vi "Set-cam-angle.vi"(2 "Rot(CAM)":dbl, 3 "Rot(rad)":dbl) -> (0 "Angle":dbl)   [LabVIEW 2011]
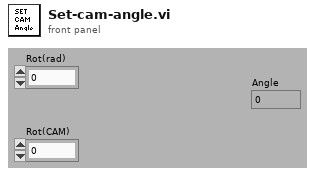
[diagram p1: front panel]
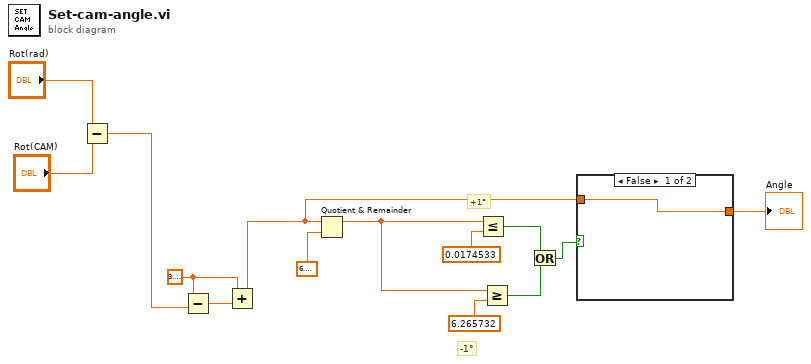
[diagram p0: block diagram]
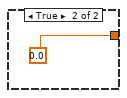
[diagram p2: hidden frame]
diagram:
  w13 = 3.141592653589793
  # "-1°"
  # "+1°"
  n1 = Subtract(x="Rot(rad)", y="Rot(CAM)") -> (x-y=w10:dbl)
  n2 = Subtract(x=w13, y=w10) -> (x-y=w14:dbl)
  n3 = Add(x=w13, y=w14) -> (x+y=w1:dbl)
  n4 = Quotient & Remainder(x=w1, y=6.283185307179586) -> (x-y*floor(x/y)=w5:dbl)  [unwired: 1 out]
  n5 = Less Or Equal?(x=w5, y=0.0174533 ("upper limit")) -> (x <= y?=w3:bool)
  n6 = Greater Or Equal?(x=w5, y=6.265732 ("upper limit")) -> (x >= y?=w4:bool)
  n7 = Or(x=w3, y=w4) -> (x .or. y?=w2:bool)
  n8 = case shown="False" w2 {
    tunnel: [w15 0.0 ("Rot(rad)")] -> w7
    tunnel: w1 -> [w15 _]
    frame False {
    }
    frame True {
    }
  }
  "Angle" <- w7
